vi "NIC Ctrl Ref FGV.vi"(2 "Network Settings Ctrl Refs":T1, 3 "FGV State":T2) -> (4 "Network Settings Ctrl Refs":T1)   [LabVIEW 2014, in "LMH-LINX.lvlib"]
uses:
  <vilib>/MakerHub/LINX/LMH-LINX.lvlib
  <vilib>/MakerHub/LINX/Private/Utilties/Target Management/Generic FGV State.ctl
  <vilib>/MakerHub/LINX/Private/Utilties/Target Management/Network Settings Ctrl Refs.ctl
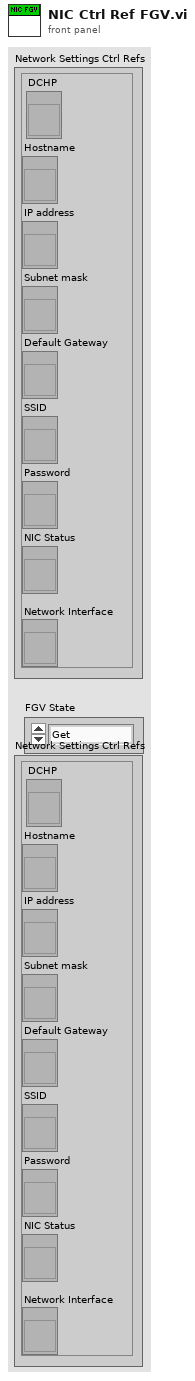
[diagram p1: front panel]
types:
  T1 = typedef "LMH-LINX.lvlib/Network Settings Ctrl Refs.ctl" = cluster{"Hostname":refnum<vi>, "IP address":refnum<vi>, "Subnet mask":refnum<vi>, "Default Gateway":refnum<vi>, "SSID":refnum<vi>, "Password":refnum<vi>, "NIC Status":refnum<vi>, "Network Interface":refnum<vi>, "DCHP":refnum<vi>}
  T2 = typedef "LMH-LINX.lvlib/Generic FGV State.ctl" = enum16{"Get", "Set"}
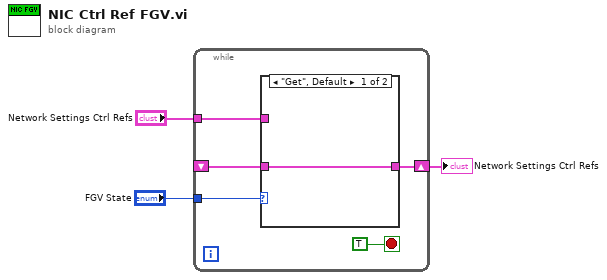
[diagram p0: block diagram]
diagram:
  n1 = while {
    tunnel: "FGV State" -> [w7]
    tunnel: "Network Settings Ctrl Refs" -> [w6]
    shift-right: [w5] -> w1
    shift-left: _ -> [w4]
    stop <- TRUE stop-if-true
    n2 = case shown="\"Get\", Default" w7 {
      tunnel: w6 -> [_ w10]
      tunnel: [w9 w10] -> w5
      tunnel: w4 -> [w9 _]
      frame "Get", Default {
      }
      frame "Set" {
      }
    }
  }
  "Network Settings Ctrl Refs" <- w1
